vi "mm_queue.vi"() -> (0 "error out":errorcluster, 3 "MM_STATE":refnum<queue>)   [LabVIEW 2013]
uses:
  main_machine/type_defs/mm_states.ctl
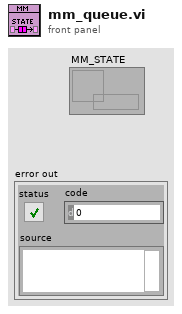
[diagram p1: front panel]
types:
  T1 = typedef "mm_states.ctl" = enum16{"STARTUP", "WAIT FOR COMMAND", "INITIALIZE INSTRUMENT", "FIND FCS FILE ", "START EXPERIMENT", "WAIT TO SAMPLE ", "DILUTE", "TAKE SAMPLE ", "EXIT"}
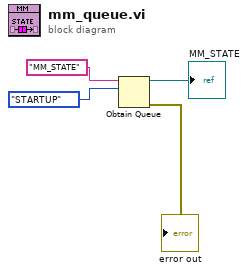
[diagram p0: block diagram]
diagram:
  n1 = Obtain Queue(name (unnamed)="MM_STATE", element data type=mm_states."STARTUP" ("Enum")) -> (queue out=→"MM_STATE":refnum<queue>, error out=→"error out":errorcluster)  [unwired: 3 in, 1 out]
